vi "UT1E3_Maquina_de_estados.vi"() -> ()   [LabVIEW 2025]
panel:
  out "a0":bool
  out "PIEZA GRUESA":dbl
  out "PIEZA DELGADA":dbl
  out "Delgada":bool
  out "Gruesa":bool
  out "a3":bool
  out "a2":bool
  out "a1":bool
  in  "STOP":bool
  in  "INICIO":bool
  in  "stop":bool
  in  "Delgada/Gruesa":bool
  # "NÚMERO DE PIEZAS"
  # "TALADRO"
  # "PARO EMERGENCIA"
  # "ALEJANDRO ALCÁNTAR SOTO\nDANIEL BONILLA DE LUNA\nURIEL EMILIANO SANTIAGO VARGAS"
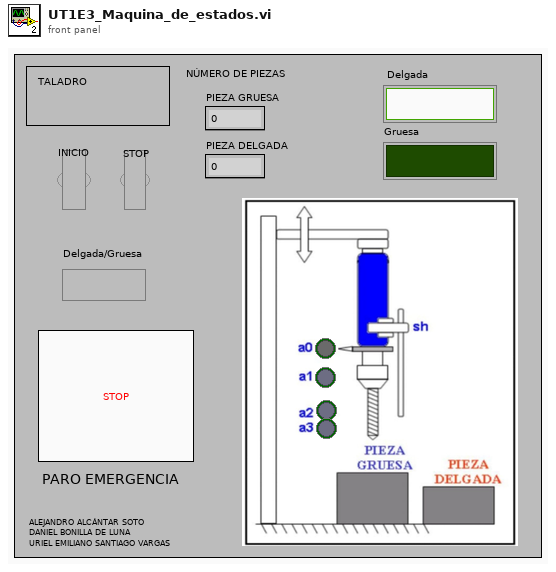
[diagram p1: front panel]
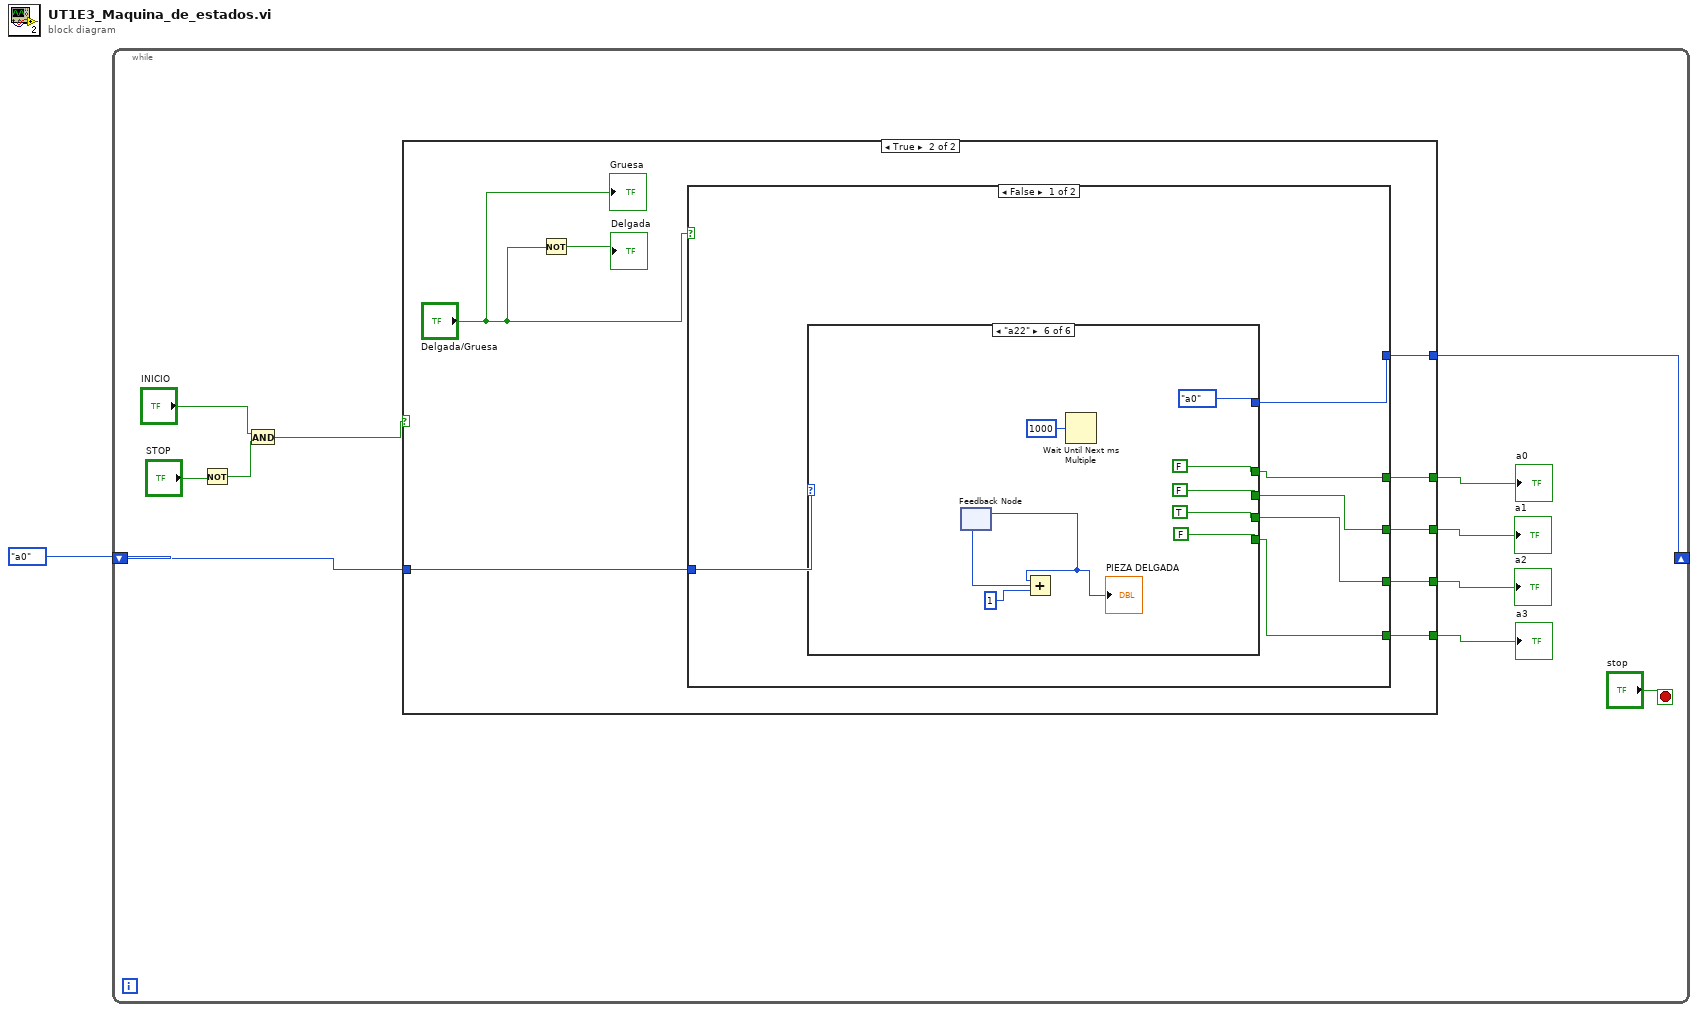
[diagram p0: block diagram]
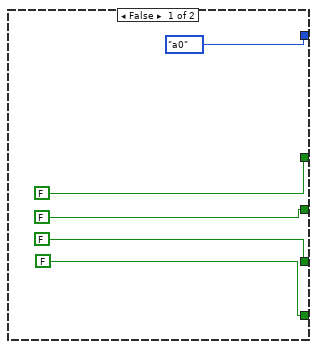
[diagram p2: hidden frame]
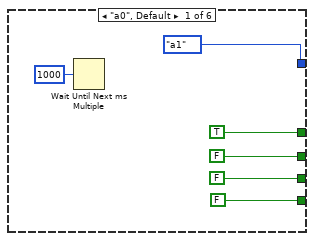
[diagram p3: hidden frame]
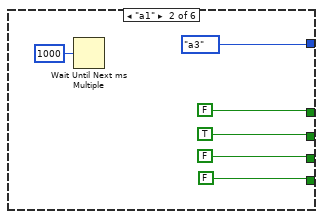
[diagram p4: hidden frame]
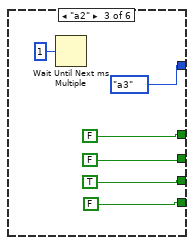
[diagram p5: hidden frame]
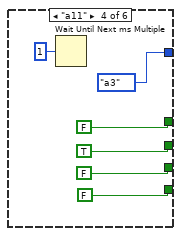
[diagram p6: hidden frame]
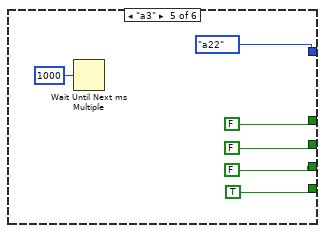
[diagram p7: hidden frame]
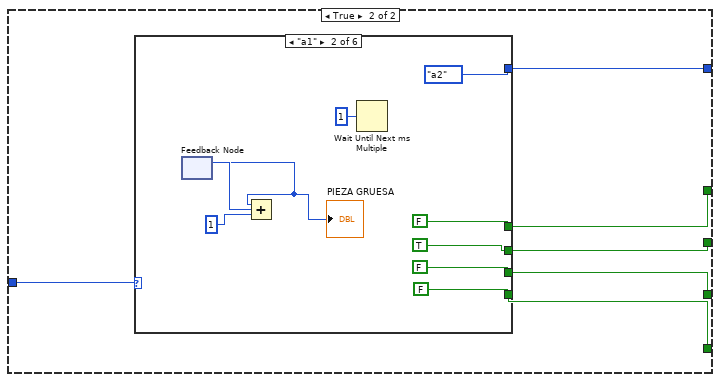
[diagram p8: hidden frame]
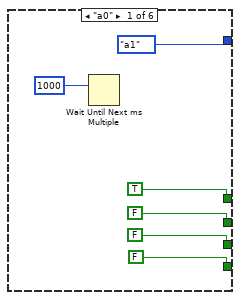
[diagram p9: hidden frame]
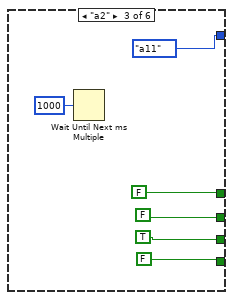
[diagram p10: hidden frame]
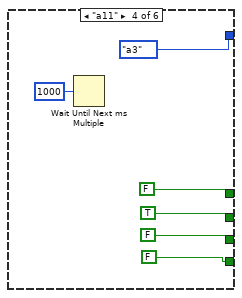
[diagram p11: hidden frame]
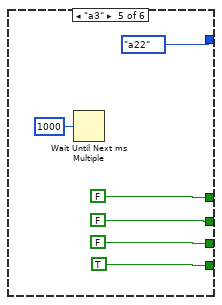
[diagram p12: hidden frame]
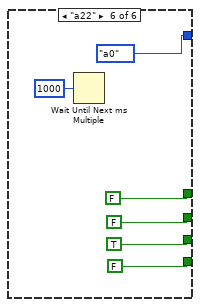
[diagram p13: hidden frame]
diagram:
  n1 = while {
    shift-right: [w3] -> _
    shift-left: enum16{"a0", "a1", "a2", "a11", "a3", "a22"}."a0" -> [w4]
    stop <- "stop" stop-if-true
    n2 = Not(x="STOP") -> (.not. x?=w9:bool)
    n3 = And(x="INICIO", y=w9) -> (x .and. y?=w2:bool)
    n4 = case shown="True" w2 {
      tunnel: [FALSE w25] -> w8
      tunnel: [FALSE w24] -> w7
      tunnel: [FALSE w23] -> w6
      tunnel: [FALSE w22] -> w5
      tunnel: w4 -> [_ w21]
      tunnel: [enum16{"a0", "a1", "a2", "a11", "a3", "a22"}."a0" w20] -> w3
      frame False {
      }
      frame True {
        n5 = Not(x="Delgada/Gruesa") -> (.not. x?=→"Delgada":bool)
        n6 = case shown="False" "Delgada/Gruesa" {
          tunnel: [w31 w71] -> w25
          tunnel: [w30 w72] -> w24
          tunnel: [w29 w73] -> w23
          tunnel: [w28 w74] -> w22
          tunnel: w21 -> [w27 w76]
          tunnel: [w26 w75] -> w20
          frame False {
            n7 = case shown="\"a22\"" w27 {
              tunnel: [enum16{"a0", "a1", "a2", "a11", "a3", "a22"}."a1" enum16{"a0", "a1", "a2", "a11", "a3", "a22"}."a3" enum16{"a0", "a1", "a2", "a11", "a3", "a22"}."a3" enum16{"a0", "a1", "a2", "a11", "a3", "a22"}."a3" enum16{"a0", "a1", "a2", "a11", "a3", "a22"}."a22" enum16{"a0", "a1", "a2", "a11", "a3", "a22"}."a0"] -> w26
              tunnel: [TRUE FALSE FALSE FALSE FALSE FALSE] -> w28
              tunnel: [FALSE TRUE FALSE TRUE FALSE FALSE] -> w29
              tunnel: [FALSE FALSE TRUE FALSE FALSE TRUE] -> w30
              tunnel: [FALSE FALSE FALSE FALSE TRUE FALSE] -> w31
              frame "a0", Default {
                n8 = Wait Until Next ms Multiple(millisecond multiple=u32 1000) -> ()  [unwired: 1 out]
              }
              frame "a1" {
                n9 = Wait Until Next ms Multiple(millisecond multiple=u32 1000) -> ()  [unwired: 1 out]
              }
              frame "a2" {
                n10 = Wait Until Next ms Multiple(millisecond multiple=u32 1) -> ()  [unwired: 1 out]
              }
              frame "a11" {
                n11 = Wait Until Next ms Multiple(millisecond multiple=u32 1) -> ()  [unwired: 1 out]
              }
              frame "a3" {
                n12 = Wait Until Next ms Multiple(millisecond multiple=u32 1000) -> ()  [unwired: 1 out]
              }
              frame "a22" {
                n13 = feedback #1() -> (w62:i32)  [unwired: 1 in]
                "PIEZA DELGADA" <- w62
                n14 = Add(x=w62, y=1) -> (x+y=w63:i32)
                n15 = feedback-in #1(w63) -> ()
                n16 = Wait Until Next ms Multiple(millisecond multiple=u32 1000) -> ()  [unwired: 1 out]
              }
            }
          }
          frame True {
            n17 = case shown="\"a1\"" w76 {
              tunnel: [enum16{"a0", "a1", "a2", "a11", "a3", "a22"}."a1" enum16{"a0", "a1", "a2", "a11", "a3", "a22"}."a2" enum16{"a0", "a1", "a2", "a11", "a3", "a22"}."a11" enum16{"a0", "a1", "a2", "a11", "a3", "a22"}."a3" enum16{"a0", "a1", "a2", "a11", "a3", "a22"}."a22" enum16{"a0", "a1", "a2", "a11", "a3", "a22"}."a0"] -> w75
              tunnel: [TRUE FALSE FALSE FALSE FALSE FALSE] -> w74
              tunnel: [FALSE TRUE FALSE TRUE FALSE FALSE] -> w73
              tunnel: [FALSE FALSE TRUE FALSE FALSE TRUE] -> w72
              tunnel: [FALSE FALSE FALSE FALSE TRUE FALSE] -> w71
              frame "a0" {
                n18 = Wait Until Next ms Multiple(millisecond multiple=u32 1000) -> ()  [unwired: 1 out]
              }
              frame "a1" {
                n19 = feedback #2() -> (w83:i32)  [unwired: 1 in]
                "PIEZA GRUESA" <- w83
                n20 = Add(x=w83, y=1) -> (x+y=w84:i32)
                n21 = feedback-in #2(w84) -> ()
                n22 = Wait Until Next ms Multiple(millisecond multiple=u32 1) -> ()  [unwired: 1 out]
              }
              frame "a2" {
                n23 = Wait Until Next ms Multiple(millisecond multiple=u32 1000) -> ()  [unwired: 1 out]
              }
              frame "a11" {
                n24 = Wait Until Next ms Multiple(millisecond multiple=u32 1000) -> ()  [unwired: 1 out]
              }
              frame "a3" {
                n25 = Wait Until Next ms Multiple(millisecond multiple=u32 1000) -> ()  [unwired: 1 out]
              }
              frame "a22" {
                n26 = Wait Until Next ms Multiple(millisecond multiple=u32 1000) -> ()  [unwired: 1 out]
              }
            }
          }
        }
        "Gruesa" <- "Delgada/Gruesa"
      }
    }
    "a0" <- w5
    "a1" <- w6
    "a2" <- w7
    "a3" <- w8
  }
